vi "Test WS Internet Echo.vi"(8 "error in (no error)":errorcluster, 11 "TestCase in":refnum<class "Test WebSockets Client.lvclass">) -> (0 "error out":errorcluster, 3 "TestCase out":refnum<class "Test WebSockets Client.lvclass">)   [LabVIEW 2013, in "Test WebSockets Client.lvclass"]
uses:
  Test WebSockets Client.lvclass
  <vilib>/addons/_JKI Toolkits/VI Tester/TestCase.llb/TestCase.lvclass
  WebSockets/WebSockets.lvlib
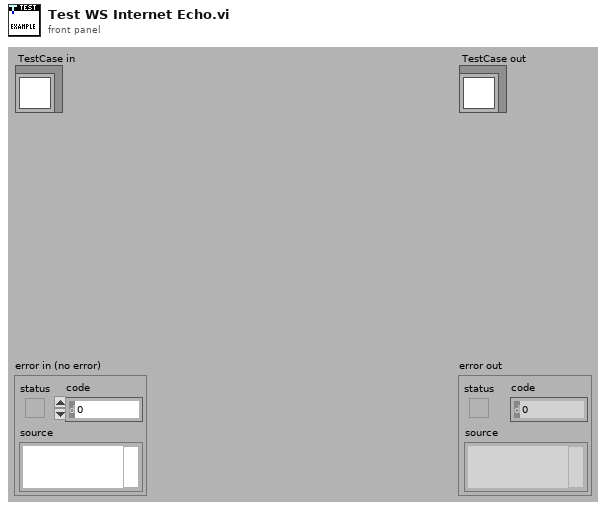
[diagram p1: front panel]
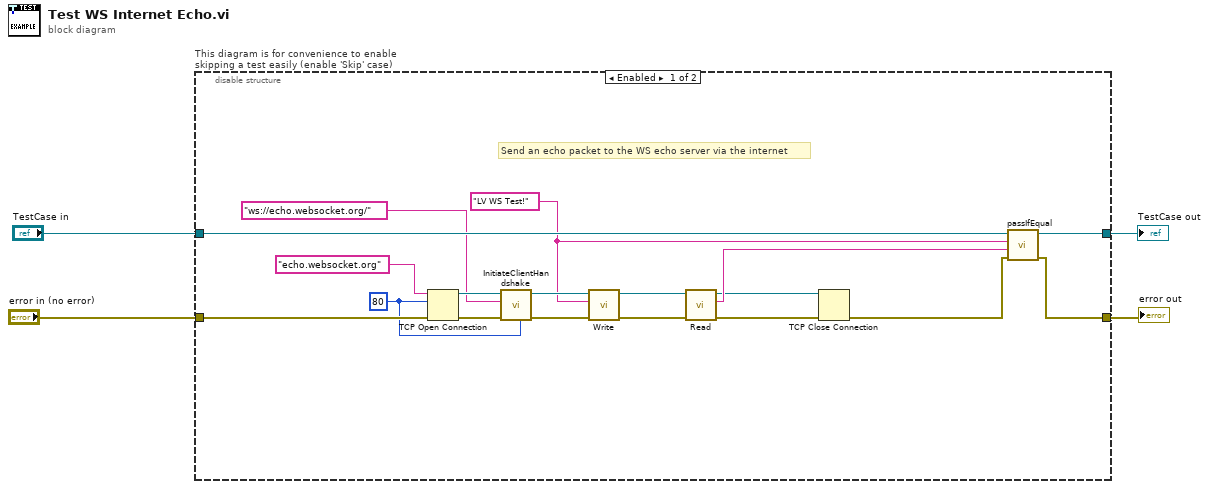
[diagram p0: block diagram]
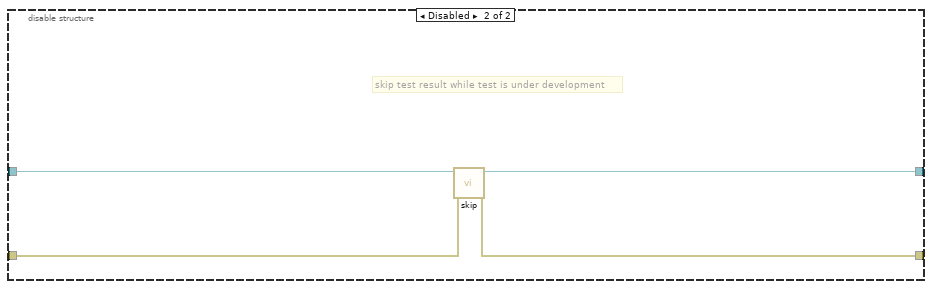
[diagram p2: hidden frame]
diagram:
  n1 = disable-structure "This diagram is for convenience to enable skipping a test easily (enable 'Skip' case)" shown="Enabled" {
    disable-tunnel: "TestCase in" -> [w21 w26]
    disable-tunnel: [w20 w24] -> w1
    disable-tunnel: [w19 w25] -> w3
    disable-tunnel: "error in (no error)" -> [w22 w23]
    frame Enabled {
      w7 = u16 80 ("remote port or service name")
      w11 = "LV WS Test!"
      # "Send an echo packet to the WS echo server via the internet"
      n2 = TCP Open Connection(address="echo.websocket.org", remote port or service name=w7, error in (no error)=w22) -> (connection ID=w18:refnum<k5>, error out=w17:errorcluster)  [unwired: 2 in]
      n3 = call "InitiateClientHandshake.vi"("remote port or service name"=w7, "error in (no error)"=w17, "request URI ('/')"="ws://echo.websocket.org/", "WebSocket Connection in"=w18) -> ("error out"=w16:errorcluster, "WebSocket Connection out"=w15:refnum<k5>)  [unwired: 5 in, 1 out]
      n4 = call "Write.vi"("error in (no error)"=w16, "Data"=w11, "WebSocket Connection in"=w15) -> ("error out"=w14:errorcluster, "WebSocket Connection out"=w13:refnum<k5>)  [unwired: 7 in]
      n5 = call "Read.vi"("error in (no error)"=w14, "WebSocket Connection in"=w13) -> ("error out"=w10:errorcluster, "Data"=w12:string, "WebSocket Connection out"=w8:refnum<k5>)  [unwired: 5 in, 2 out]
      n6 = TCP Close Connection(connection ID=w8, error in (no error)=w10) -> (error out=w9:errorcluster)  [unwired: 1 in, 1 out]
      n7 = call-dynamic "passIfEqual.vi"("error in (no error)"=w9, "y"=w12, "x"=w11, "TestCase in"=w21) -> ("error out"=w19:errorcluster, "TestCase out"=w20:refnum<class "Test WebSockets Client.lvclass">)  [unwired: 6 in]
    }
    frame Disabled {
      # "skip test result while test is under development"
      n8 = call <vilib>:"skip.vi"("error in (no error)"=w23, "TestCase in"=w26) -> ("error out"=w25:errorcluster, "TestCase out"=w24:refnum<class "Test WebSockets Client.lvclass">)  [unwired: 8 in]
    }
  }
  "error out" <- w3
  "TestCase out" <- w1
